vi "Main_Test.vi"() -> ()   [LabVIEW 2018]
panel:
  out "Modele Name":string
  out "Status":bool
  in  "Serial Number":string
  out "OperatorID":string
  out "Recipe File":string="C:/Valeo/MicrophoneTest/ME79_limits.csv"
  out "Progress":u8(slide) scale=0.0..100.0
  out "TestData":i32(listbox)
  # "Valeo.com"
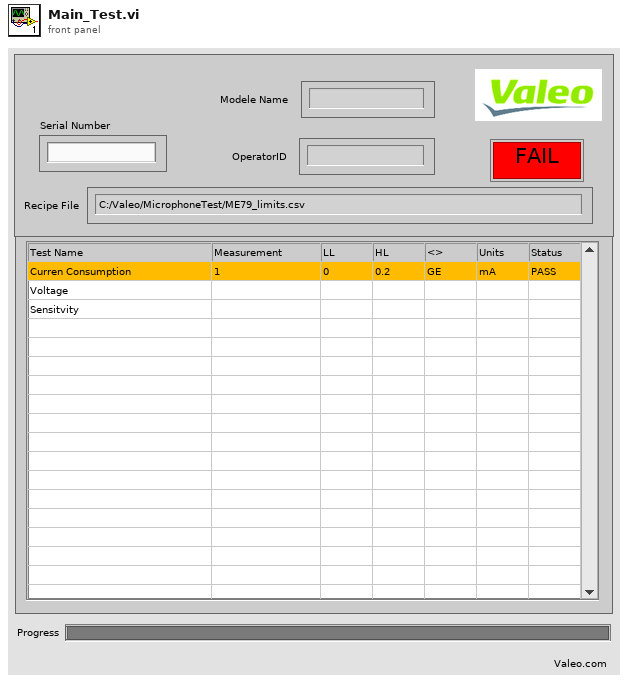
[diagram p1: front panel]
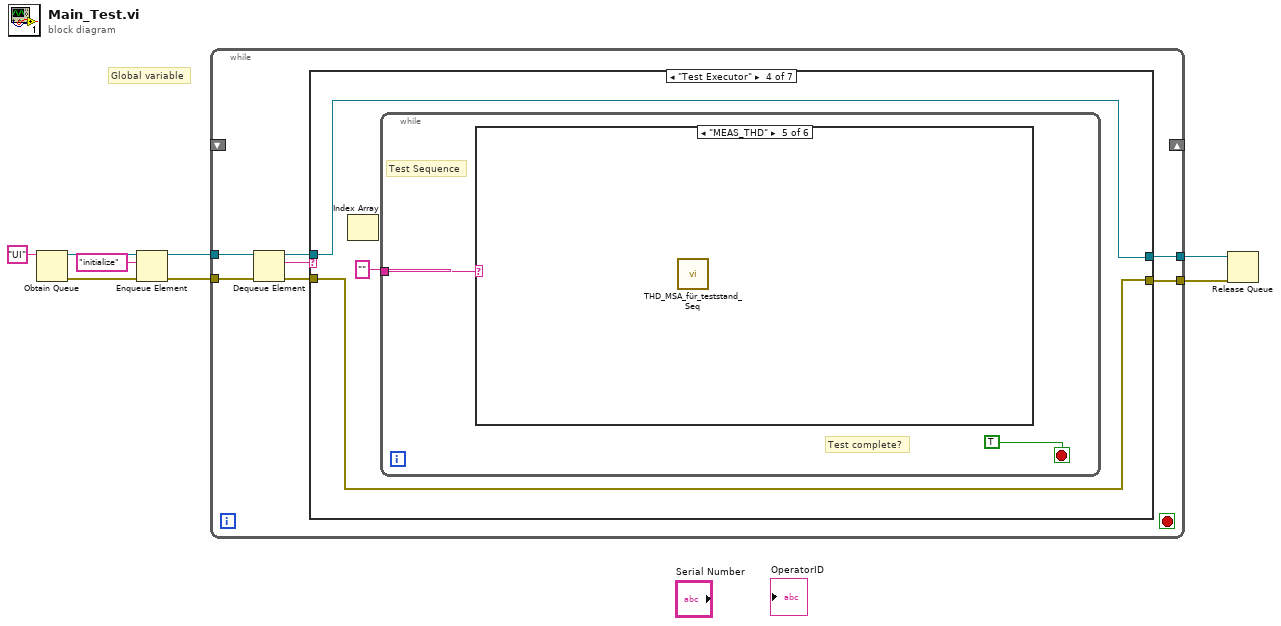
[diagram p0: block diagram]
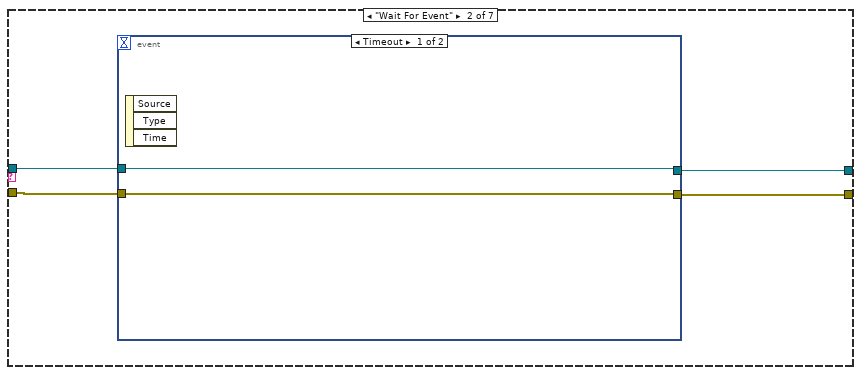
[diagram p3: hidden frame]
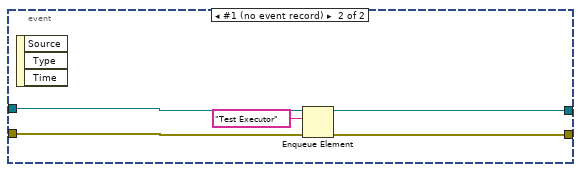
[diagram p4: hidden frame]
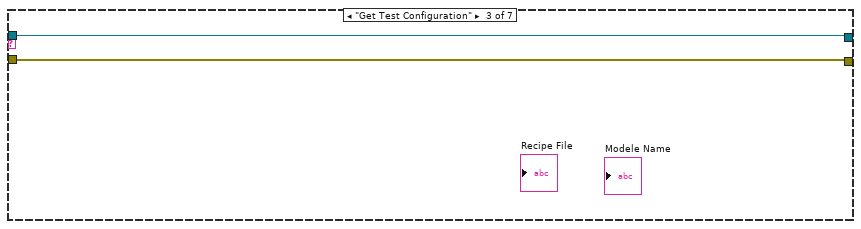
[diagram p5: hidden frame]
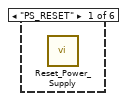
[diagram p6: hidden frame]
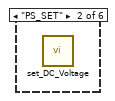
[diagram p7: hidden frame]
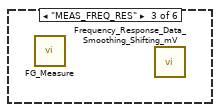
[diagram p8: hidden frame]
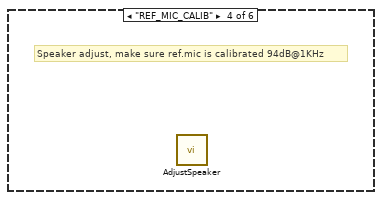
[diagram p9: hidden frame]
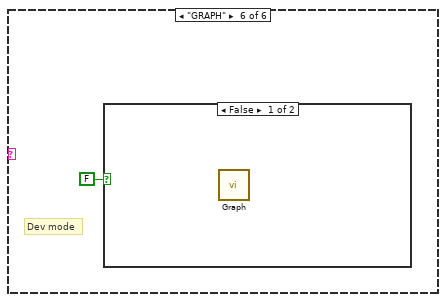
[diagram p10: hidden frame]
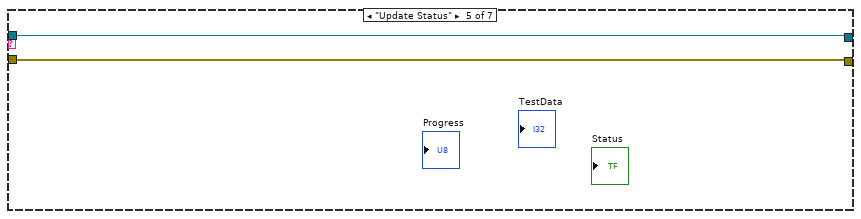
[diagram p12: hidden frame]
diagram:
  # "Global variable"
  n1 = Obtain Queue(name (unnamed)="UI") -> (queue out=w5:refnum<queue>, error out=w8:errorcluster)  [unwired: 4 in, 1 out]
  n2 = Enqueue Element(queue=w5, element="initialize", error in (no error)=w8) -> (queue out=w3:refnum<queue>, error out=w7:errorcluster)  [unwired: 1 in, 1 out]
  n3 = while {
    tunnel: w7 -> [w15]
    tunnel: w3 -> [w11]
    tunnel: [w10] -> w2
    tunnel: [w9] -> w1
    shift-right: _ -> [_]
    shift-left: _ -> [_]
    stop <- _ stop-if-true
    n4 = Dequeue Element(queue=w11, error in (no error)=w15) -> (queue out=w12:refnum<queue>, element=w13:string, error out=w14:errorcluster)  [unwired: 1 in, 1 out]
    n5 = case shown="\"Test Executor\"" w13 {
      tunnel: w14 -> [w16 w20 w29 w32 w37 w39 w41]
      tunnel: w12 -> [w17 w21 w30 w33 w38 w40 w42]
      tunnel: [w16 w19 w29 w32 w37 w39 w41] -> w10
      tunnel: [w17 w18 w30 w33 w38 w40 w42] -> w9
      frame "Initialize", Default {
      }
      frame "Wait For Event" {
        n6 = event shown="[0] Timeout" {
          selector: _ -> [_ _]
          dyn-events: _ -> [_ _]
          timeout: _ -> [_ _]
          tunnel: w21 -> [w23 w28]
          tunnel: w20 -> [w22 w27]
          tunnel: [w22 w25] -> w19
          tunnel: [w23 w24] -> w18
          event Timeout {
            n7 = event-data() -> ()  [unwired: 1 in, 3 out]
          }
          event #1 (no event record) {
            n8 = event-data() -> ()  [unwired: 1 in, 3 out]
            n9 = Enqueue Element(queue=w28, element="Test Executor", error in (no error)=w27) -> (queue out=w24:refnum<queue>, error out=w25:errorcluster)  [unwired: 1 in, 1 out]
          }
        }
      }
      frame "Get Test Configuration" {
      }
      frame "Test Executor" {
        n10 = Index Array() -> ()  [unwired: 2 in, 1 out]
        n11 = while {
          tunnel: "" -> [w35]
          stop <- TRUE stop-if-true
          # "Test complete?"
          # "Test Sequence"
          n12 = case shown="\"MEAS_THD\"" w35 {
            frame "PS_RESET" {
              n13 = call "Reset_Power_Supply.vi"() -> ()  [unwired: 11 in, 1 out]
            }
            frame "PS_SET" {
              n14 = call "set_DC_Voltage.vi"() -> ()  [unwired: 8 in, 4 out]
            }
            frame "MEAS_FREQ_RES" {
              n15 = call "FG_Measure.vi"() -> ()  [unwired: 10 in, 6 out]
              n16 = call "Frequency_Response_Data_Smoothing_Shifting_mV.vi"() -> ()  [unwired: 19 in, 1 out]
            }
            frame "REF_MIC_CALIB" {
              # "Speaker adjust, make sure ref.mic is calibrated 94dB@1KHz"
              n17 = call "AdjustSpeaker.vi"() -> ()  [unwired: 9 in, 3 out]
            }
            frame "MEAS_THD" {
              n18 = call "THD_MSA_für_teststand_Seq.vi"() -> ()  [unwired: 9 in, 3 out]
            }
            frame "GRAPH" {
              # "Dev mode"
              n19 = case shown="False" FALSE {
                frame False {
                  n20 = call "Graph.vi"() -> ()  [unwired: 10 in, 2 out]
                }
                frame True {
                }
              }
            }
          }
        }
      }
      frame "Update Status" {
      }
      frame "Load limits" {
      }
      frame "Clean Up" {
      }
    }
  }
  n21 = Release Queue(queue=w1, error in (no error)=w2) -> ()  [unwired: 1 in, 3 out]
